vi "Update Value.vi"(6 "Time":dbl, 8 "error in (no error)":errorcluster, 11 "ButtonControl in":refnum<class "DigitalButtonControl.lvclass">) -> (0 "error out":errorcluster, 1 "Update":bool, 2 "Value":variant, 3 "ButtonControl out":refnum<class "DigitalButtonControl.lvclass">)   [LabVIEW 2020, in "VolatusGUIElements.lvlib" / "DigitalButtonControl.lvclass"]
uses:
  DigitalButtonControl.lvclass
  DigitalButtonControl.lvclass/DigitalButtonControl.ctl
  lv-vecto/Vecto/Channel/Channel.lvclass/Channel.ctl
  lv-vecto/Vecto/Group/Value by Index.vi
  lv-vecto/Vecto/Channel/Channel.lvclass
  VolatusGUIElements.lvlib
  lv-vecto/Vecto/Vecto.lvlib
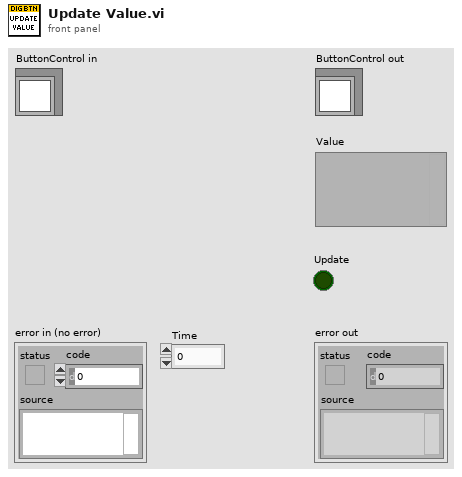
[diagram p1: front panel]
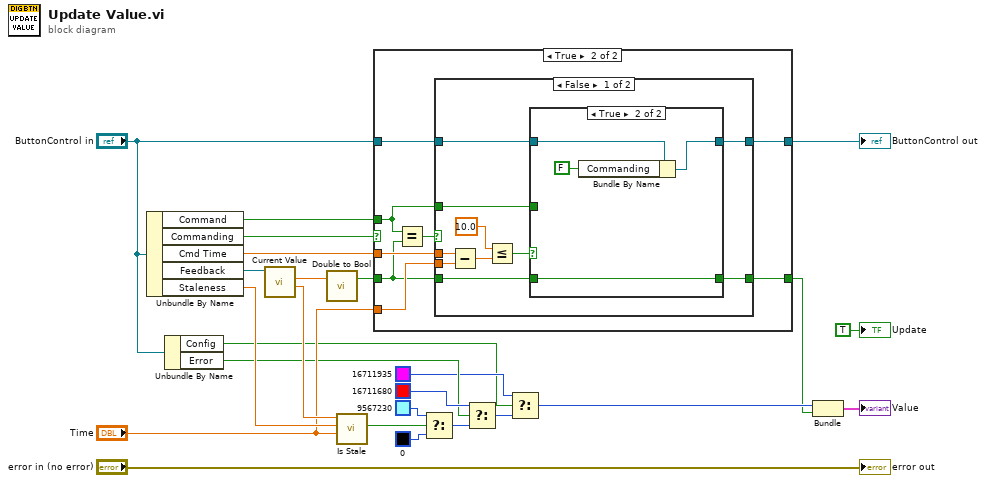
[diagram p0: block diagram]
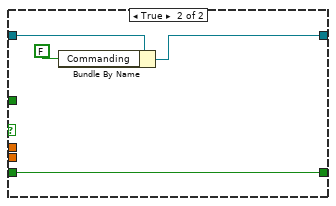
[diagram p4: hidden frame]
diagram:
  n1 = Unbundle By Name("ButtonControl in") -> ("Command"=w7:bool, "Commanding"=w21:bool, "Cmd Time"=w19:dbl, "Feedback"=w24:refnum<class "Channel.lvclass">, "Staleness"=w22:dbl)
  n2 = Unbundle By Name("ButtonControl in") -> ("Config"=w8:bool, "Error"=w11:bool)
  n3 = call "Current Value.vi"("Channel in"=w24) -> ("Timestamp"=w23:dbl, "Scaled"=w20:dbl)  [unwired: 6 in, 3 out]
  n4 = call "Double to Bool.vi"("Double"=w20) -> ("Bool"=w18:bool)  [unwired: 2 in]
  n5 = call "Is Stale.vi"("Time"="Time", "Staleness"=w22, "Timestamp"=w23) -> ("Stale"=w16:bool)  [unwired: 8 in]
  n6 = case shown="True" w21 {
    tunnel: w18 -> [w27 w32]
    tunnel: w19 -> [_ w35]
    tunnel: "Time" -> [_ w34]
    tunnel: w7 -> [_ w28]
    tunnel: "ButtonControl in" -> [w26 w31]
    tunnel: [w26 w30] -> w5
    tunnel: [w27 w29] -> w3
    frame False {
    }
    frame True {
      n7 = Equal?(x=w28, y=w32) -> (x = y?=w33:bool)
      n8 = case shown="False" w33 {
        tunnel: w35 -> [w45 _]
        tunnel: w34 -> [w44 _]
        tunnel: w32 -> [w38 w52]
        tunnel: w31 -> [w40 w55]
        tunnel: [w39 w53] -> w30
        tunnel: [w36 w52] -> w29
        tunnel: w28 -> [w37 _]
        frame False {
          n9 = Subtract(x=w45, y=w44) -> (x-y=w43:dbl)
          n10 = Less Or Equal?(x=10.0, y=w43) -> (x <= y?=w41:bool)
          n11 = case shown="True" w41 {
            tunnel: w40 -> [w46 w51]
            tunnel: [w46 w49] -> w39
            tunnel: w38 -> [_ w48]
            tunnel: w37 -> [w47 _]
            tunnel: [w47 w48] -> w36
            frame False {
            }
            frame True {
              n12 = Bundle By Name(cluster=w51, "Commanding"=FALSE) -> (w49:refnum<class "DigitalButtonControl.lvclass">)
            }
          }
        }
        frame True {
          n13 = Bundle By Name(cluster=w55, "Commanding"=FALSE) -> (w53:refnum<class "DigitalButtonControl.lvclass">)
        }
      }
    }
  }
  "ButtonControl out" <- w5
  n14 = Select(t=u32 9567230, s=w16, f=u32 0) -> (s? t:f=w13:u32)
  n15 = Select(t=u32 16711680, s=w11, f=w13) -> (s? t:f=w10:u32)
  n16 = Select(t=u32 16711935, s=w8, f=w10) -> (s? t:f=w4:u32)
  n17 = Bundle(w4, "Bool"=w3) -> (→"Value":cluster{u32, "Bool":bool})  [unwired: 1 in]
  "error out" <- "error in (no error)"
  "Update" <- TRUE ("Update")
